vi "TCP Read (SubVI).vi"(0 "Status in":refnum<vi>, 7 "Value":refnum<k5>, 11 "error in (no error)":errorcluster) -> (1 "Drv":u8, 2 "opcode R":u32 format="%.0x", 3 "Csum R":u16, 4 "Rx data tmp":u8[](array[numeric]) format="%.0x", 6 "Destination R":u32, 8 "CSum":bool, 10 "Drv Array":u8[](array[numeric]), 12 "Source  R":u32, 13 "MsgCnt R":u32, 14 "Read array":u8[](array[numeric]) format="%x", 15 "error out":errorcluster)   [LabVIEW 2017]
panel:
  out "Read array 2":u8[](array[numeric]) format="%x"
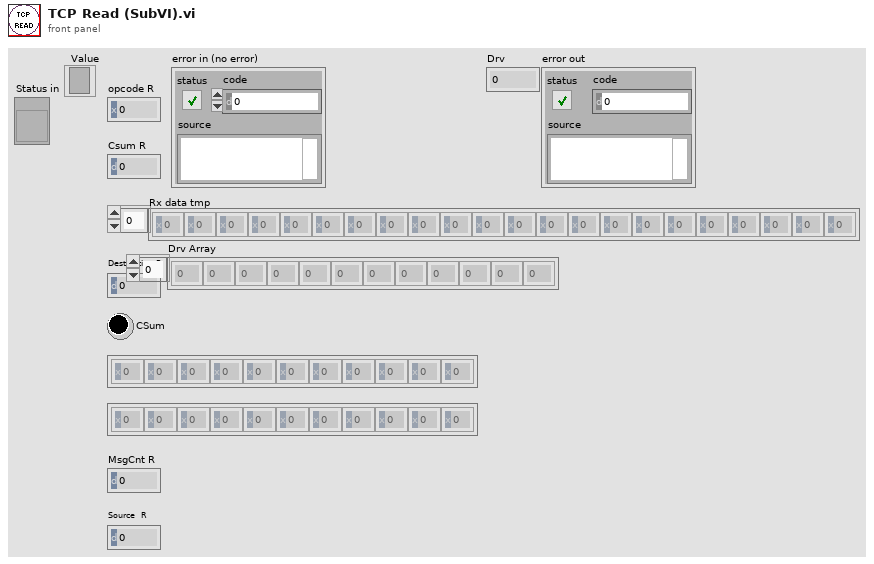
[diagram p1: front panel]
types:
  T1 = enum16{"Standard", "Buffered", "CRLF", "Immediate"}
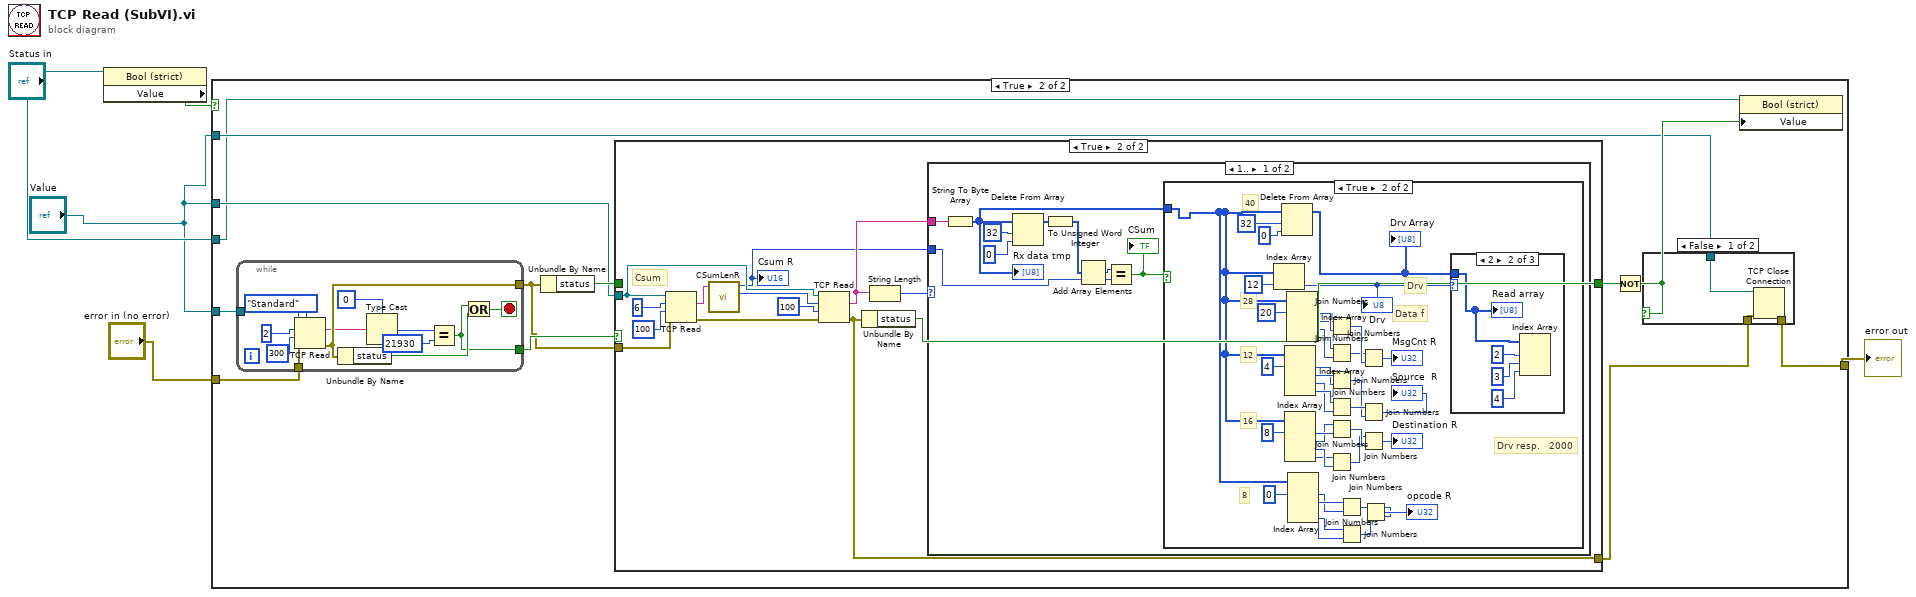
[diagram p0: block diagram]
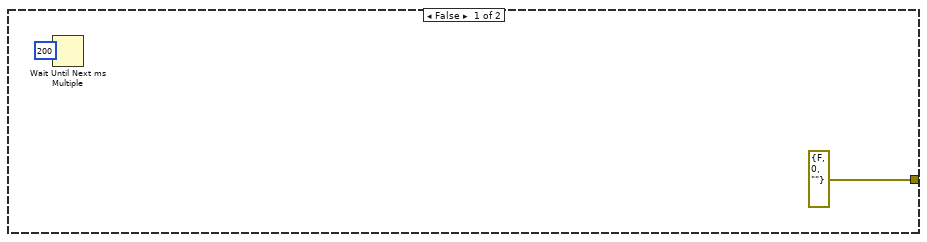
[diagram p2: hidden frame]
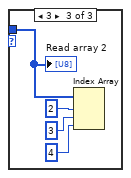
[diagram p7: hidden frame]
diagram:
  n1 = property class="Bool (strict)"(reference="Status in") -> ("Value"=w5:bool)  [unwired: 1 in, 2 out]
  n2 = case shown="True" w5 {
    tunnel: [errorcluster {"status"=FALSE, "code"=0, "source"=""} ("warning out") w13] -> w3
    tunnel: "Value" -> [_ w12]
    tunnel: "Value" -> [_ w11]
    tunnel: "Value" -> [_ w10]
    tunnel: "Status in" -> [_ w9]
    tunnel: "error in (no error)" -> [_ w8]
    frame False {
      n3 = Wait Until Next ms Multiple(millisecond multiple=u32 200) -> ()  [unwired: 1 out]
    }
    frame True {
      n4 = while {
        tunnel: [w104] -> w15
        tunnel: [w101] -> w19
        tunnel: w11 -> [w95]
        tunnel: w8 -> [w94]
        stop <- w102 stop-if-true
        n5 = TCP Read(connection ID=w95, bytes to read=2, error in (no error)=w94, 7:T1."Standard" ("mode (standard)"), 9:300) -> (data out=w99:string, error out=w104:errorcluster)  [unwired: 1 out]
        n6 = Unbundle By Name(w104) -> ("status"=w103:bool)
        n7 = Type Cast(type=u16 0 ("y"), x=w99) -> (*(type *) &x=w97:u16)
        n8 = Equal?(x=w97, y=u16 21930) -> (x = y?=w101:bool)
        n9 = Or(x=w101, y=w103) -> (x .or. y?=w102:bool)
      }
      n10 = Unbundle By Name(w15) -> ("status"=w16:bool)
      n11 = case shown="True" w19 {
        tunnel: w12 -> [_ w35]
        tunnel: [w25 w31] -> w18
        tunnel: w16 -> [w25 _]
        tunnel: w15 -> [w24 w27]
        tunnel: [w24 w26] -> w14
        frame False {
        }
        frame True {
          # "Csum"
          n12 = TCP Read(connection ID=w35, bytes to read=6, error in (no error)=w27, 9:100) -> (data out=w30:string, error out=w32:errorcluster)  [unwired: 1 in, 1 out]
          n13 = call "CSumLenR.vi"("data in"=w30) -> ("CSum"=w28:u16, "Len"=w29:i32)  [unwired: 8 in]
          "Csum R" <- w28
          n14 = TCP Read(connection ID=w35, bytes to read=w29, error in (no error)=w32, 9:100) -> (data out=w33:string, error out=w26:errorcluster)  [unwired: 1 in, 1 out]
          n15 = Unbundle By Name(w26) -> ("status"=w31:bool)
          n16 = String Length(string=w33) -> (length=w38:i32)
          n17 = case shown="1.." w38 {
            tunnel: w33 -> [w47 _]
            tunnel: w28 -> [w44 _]
            frame 1.. {
              n18 = String To Byte Array(string=w47) -> (unsigned byte array=w41:u8[])
              "Rx data tmp" <- w41
              n19 = Delete From Array(array=w41, length=32, index=0) -> (array with subset deleted=w40:u8[])  [unwired: 1 out]
              n20 = To Unsigned Word Integer(number=w40) -> (unsigned 16bit integer=w46:u16[])
              n21 = Add Array Elements(numeric array=w46) -> (sum=w45:u16)
              n22 = Equal?(x=w45, y=w44) -> (x = y?=w43:bool)
              "CSum" <- w43
              n23 = case shown="True" w43 {
                tunnel: w41 -> [_ w48]
                frame False {
                }
                frame True {
                  # "Drv resp.  \t2000"
                  # "Data f"
                  # "Drv"
                  # "8"
                  # "16"
                  # "12"
                  # "28"
                  # "40"
                  n24 = Index Array(array=w48, index=12) -> (element=w85:u8)
                  "Drv" <- w85
                  n25 = Delete From Array(array=w48, length=32, index=0) -> (array with subset deleted=w84:u8[])  [unwired: 1 out]
                  "Drv Array" <- w84
                  n26 = Index Array(array=w48, index #1=4 ("index")) -> (element #1=w68:u8, element #2=w69:u8, element #3=w70:u8, element #4=w71:u8)  [unwired: 3 in]
                  n27 = Index Array(array=w48, index #1=8 ("index")) -> (element #1=w79:u8, element #2=w78:u8, element #3=w77:u8, element #4=w76:u8)  [unwired: 3 in]
                  n28 = Index Array(array=w48, index #1=20 ("index")) -> (element #1=w67:u8, element #2=w66:u8, element #3=w65:u8, element #4=w64:u8)  [unwired: 3 in]
                  n29 = Index Array(array=w48, index #1=0 ("index")) -> (element #1=w56:u8, element #2=w57:u8, element #3=w58:u8, element #4=w59:u8)  [unwired: 3 in]
                  n30 = Join Numbers(hi=w66, lo=w67) -> ((hi.lo)=w63:u16)
                  n31 = Join Numbers(hi=w64, lo=w65) -> ((hi.lo)=w62:u16)
                  n32 = Join Numbers(hi=w69, lo=w68) -> ((hi.lo)=w72:u16)
                  n33 = Join Numbers(hi=w71, lo=w70) -> ((hi.lo)=w73:u16)
                  n34 = Join Numbers(hi=w78, lo=w79) -> ((hi.lo)=w75:u16)
                  n35 = Join Numbers(hi=w76, lo=w77) -> ((hi.lo)=w74:u16)
                  n36 = Join Numbers(hi=w57, lo=w56) -> ((hi.lo)=w60:u16)
                  n37 = Join Numbers(hi=w59, lo=w58) -> ((hi.lo)=w61:u16)
                  n38 = Join Numbers(hi=w62, lo=w63) -> ((hi.lo)=→"MsgCnt R":u32)
                  n39 = Join Numbers(hi=w73, lo=w72) -> ((hi.lo)=→"Source  R":u32)
                  n40 = Join Numbers(hi=w74, lo=w75) -> ((hi.lo)=→"Destination R":u32)
                  n41 = Join Numbers(hi=w61, lo=w60) -> ((hi.lo)=→"opcode R":u32)
                  n42 = case shown="2" w85 {
                    tunnel: w84 -> [_ w87 w91]
                    frame 0, Default {
                    }
                    frame 2 {
                      n43 = Index Array(array=w87, index #1=2 ("index"), index #2=3 ("index"), index #3=4 ("index")) -> ()  [unwired: 3 out]
                      "Read array" <- w87
                    }
                    frame 3 {
                      n44 = Index Array(array=w91, index #1=2 ("index"), index #2=3 ("index"), index #3=4 ("index")) -> ()  [unwired: 3 out]
                      "Read array 2" <- w91
                    }
                  }
                }
              }
            }
            frame ..0 {
            }
          }
        }
      }
      n45 = Not(x=w18) -> (.not. x?=w17:bool)
      n46 = case shown="False" w17 {
        tunnel: w14 -> [w22 w23]
        tunnel: [w21 w23] -> w13
        tunnel: w10 -> [w20 _]
        frame False {
          n47 = TCP Close Connection(connection ID=w20, error in (no error)=w22) -> (error out=w21:errorcluster)  [unwired: 1 in, 1 out]
        }
        frame True {
        }
      }
      n48 = property class="Bool (strict)"(reference=w9, "Value"=w17) -> ()  [unwired: 1 in, 2 out]
    }
  }
  "error out" <- w3
